vi "zad1.vi"(8 "error in (no error)":errorcluster, 11 "Numeric":dbl) -> (0 "error out":errorcluster, 3 "Array":dbl[](array[numeric]))   [LabVIEW 2017]
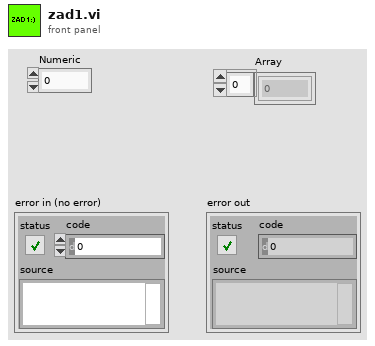
[diagram p1: front panel]
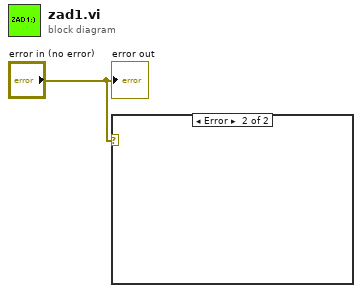
[diagram p0: block diagram]
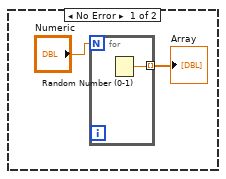
[diagram p2: hidden frame]
diagram:
  n1 = case shown="Error" "error in (no error)" {
    frame No Error {
      n2 = for {
        N: "Numeric" -> [_]
        tunnel: [w4] -> w3 mode=indexing
        n3 = Random Number (0-1)() -> (number: 0 to 1=w4:dbl)
      }
      "Array" <- w3
    }
    frame Error {
    }
  }
  "error out" <- "error in (no error)"
